vi "Set Voltage Unit.vi"(8 "error in (no error)":errorcluster, 9 "Volt Unit (VPP)":T1, 10 "Channel (0: Channel 1)":T2 items=["Channel 1", "Channel 2"], 11 "VISA resource name":refnum<visa-resource-name>) -> (0 "error out":errorcluster, 3 "VISA resource name out":refnum<visa-resource-name>)   [LabVIEW 2012, in "Tektronix AFG 3000 Series.lvlib"]
doc: "Sets the units used when setting the voltage amplitude of a Tektronix AFG 3000 series function generator. (Does not affect the offest, high, or low voltage commands.)"
uses:
  Tektronix AFG 3000 Series.lvlib
  controls.llb/Channel.ctl
  controls.llb/Volt Unit.ctl
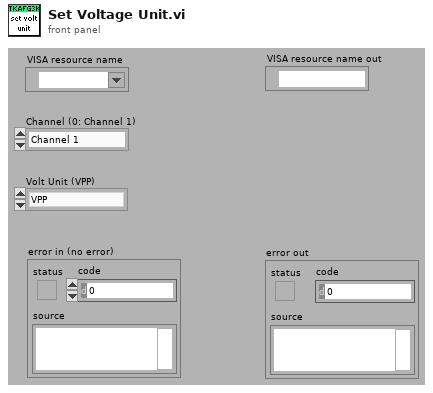
[diagram p1: front panel]
types:
  T1 = typedef "Volt Unit.ctl" = enum16{"VPP", "VRMS", "DBM"}
  T2 = typedef "Channel.ctl" = u16
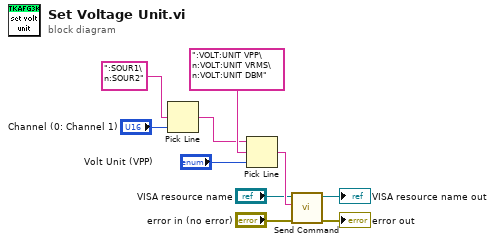
[diagram p0: block diagram]
diagram:
  n1 = Pick Line(multi-line string=":SOUR1\n:SOUR2", line index="Channel (0: Channel 1)") -> (output string=w7:string)  [unwired: 1 out]
  n2 = Pick Line(string ("")=w7, multi-line string=":VOLT:UNIT VPP\n:VOLT:UNIT VRMS\n:VOLT:UNIT DBM", line index="Volt Unit (VPP)") -> (output string=w6:string)
  n3 = call "Send Command.vi"("error in (no error)"="error in (no error)", "write buffer"=w6, "VISA resource name"="VISA resource name") -> ("error out"=→"error out":errorcluster, "VISA resource name out"=→"VISA resource name out":refnum<visa-resource-name>)  [unwired: 7 out]
